vi "m1m3_getEvent_PowerSupplyStatus.vi"(8 "error in (no error)":errorcluster, 11 "logevent_PowerSupplyStatus_Ctl":T1) -> (0 "error out":errorcluster, 2 "function return":i32, 3 "logevent_PowerSupplyStatus_Ctl out":T1)   [LabVIEW 2016, in "SALLV_m1m3.lvlib"]
doc: "int m1m3_shm_getEvent_PowerSupplyStatusLV(m1m3_logevent_PowerSupplyStatusLV *logevent_PowerSupplyStatus_Ctl );"
uses:
  SALLV_m1m3.lvlib
  DataTypes/logevent_PowerSupplyStatus.ctl
  SALLV_m1m3.so
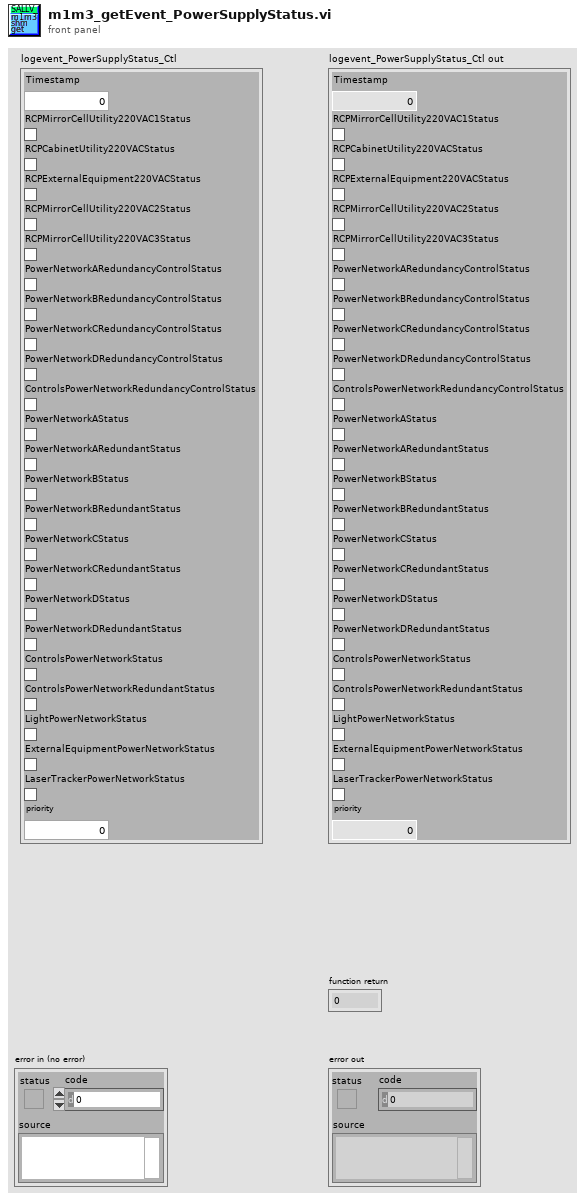
[diagram p1: front panel]
types:
  T1 = typedef "SALLV_m1m3.lvlib/logevent_PowerSupplyStatus.ctl" = cluster{"Timestamp":dbl, "RCPMirrorCellUtility220VAC1Status":bool, "RCPCabinetUtility220VACStatus":bool, "RCPExternalEquipment220VACStatus":bool, "RCPMirrorCellUtility220VAC2Status":bool, "RCPMirrorCellUtility220VAC3Status":bool, "PowerNetworkARedundancyControlStatus":bool, "PowerNetworkBRedundancyControlStatus":bool, "PowerNetworkCRedundancyControlStatus":bool, "PowerNetworkDRedundancyControlStatus":bool, "ControlsPowerNetworkRedundancyControlStatus":bool, "PowerNetworkAStatus":bool, "PowerNetworkARedundantStatus":bool, "PowerNetworkBStatus":bool, "PowerNetworkBRedundantStatus":bool, "PowerNetworkCStatus":bool, "PowerNetworkCRedundantStatus":bool, "PowerNetworkDStatus":bool, "PowerNetworkDRedundantStatus":bool, "ControlsPowerNetworkStatus":bool, "ControlsPowerNetworkRedundantStatus":bool, "LightPowerNetworkStatus":bool, "ExternalEquipmentPowerNetworkStatus":bool, "LaserTrackerPowerNetworkStatus":bool, "priority":i32}
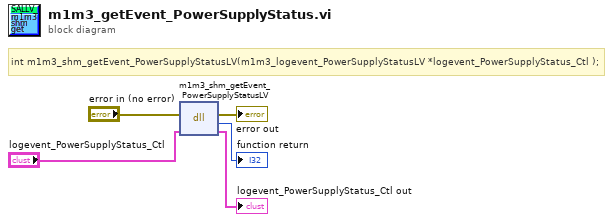
[diagram p0: block diagram]
diagram:
  # "int m1m3_shm_getEvent_PowerSupplyStatusLV(m1m3_logevent_PowerSupplyStatusLV *logevent_PowerSupplyStatus_Ctl );"
  n1 = dll-call lib="opt/CODE/SALLV_m1m3/SALLV_m1m3.*" fn="m1m3_shm_getEvent_PowerSupplyStatusLV"(error in="error in (no error)", "logevent_PowerSupplyStatus_Ctl"="logevent_PowerSupplyStatus_Ctl") -> (error out=→"error out":errorcluster, →"function return":i32, "logevent_PowerSupplyStatus_Ctl"=→"logevent_PowerSupplyStatus_Ctl out":T1)  [unwired: 2 in, 1 out]
